vi "U3 Create Frequency Output Lists.vi"() -> (1 "Period List":dbl[][](array[numeric]) format="%.6f", 2 "Frequency List":dbl[][](array[numeric]) format="%.6f")   [LabVIEW 2021]
panel:
  # "Creates 2D arrays which are lists of all the frequency/period\noptions for the Frequency Output timer mode 7.  Takes 10-15\nseconds to run on a typical PC.\n\nFrequency/Period, Base Clock, Divisor, Timer Value"
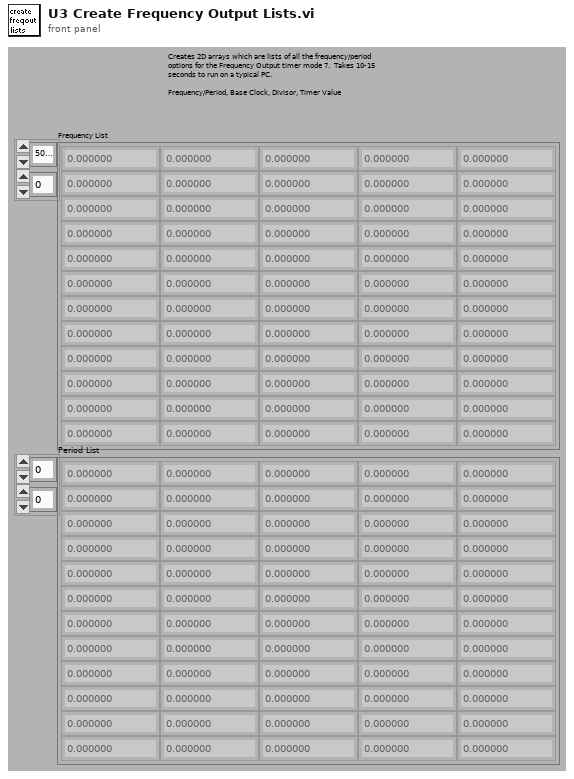
[diagram p1: front panel]
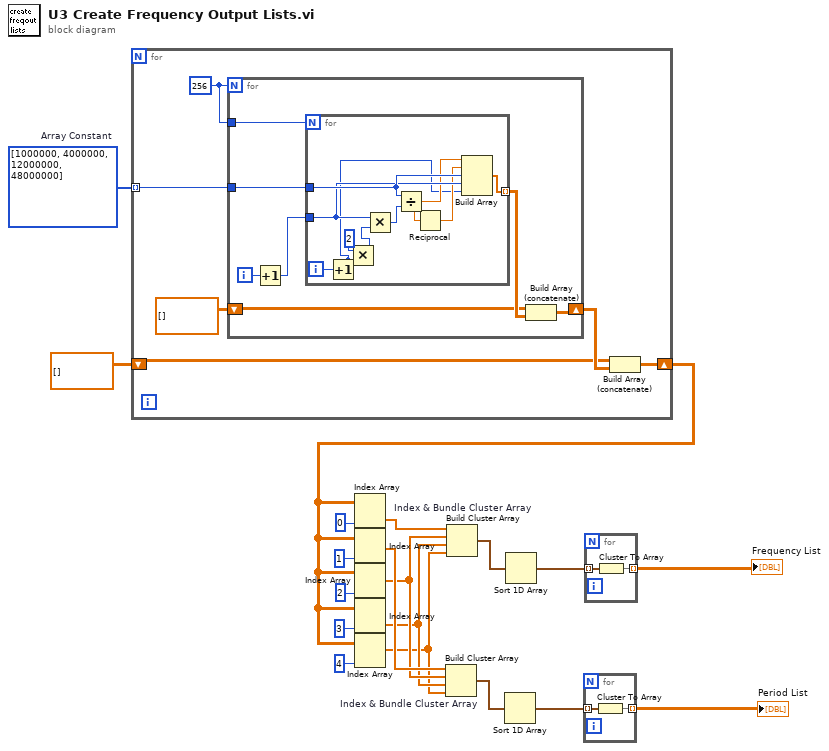
[diagram p0: block diagram]
diagram:
  w17 = i32[] [1000000, 4000000, 12000000, 48000000]  # Array Constant
  n1 = for {
    tunnel: w17 -> [w25] mode=indexing
    shift-right: [w21] -> w8
    shift-left: dbl[][] [] -> [w22]
    w24 = 256
    n2 = for {
      N: w24 -> [_]
      tunnel: w25 -> [w32]
      tunnel: w24 -> [w31]
      shift-right: [w26] -> w23
      shift-left: dbl[][] [] -> [w27]
      i -> [w30]
      n3 = Increment(x=w30) -> (x+1=w29:i32)
      n4 = for {
        N: w31 -> [_]
        tunnel: w32 -> [w40]
        tunnel: w29 -> [w39]
        tunnel: [w38] -> w28 mode=indexing
        i -> [w42]
        n5 = Increment(x=w42) -> (x+1=w33:i32)
        n6 = Multiply(x=2, y=w33) -> (x*y=w34:i32)
        n7 = Multiply(x=w39, y=w34) -> (x*y=w41:i32)
        n8 = Divide(x=w40, y=w41) -> (x/y=w36:dbl)
        n9 = Reciprocal(x=w36) -> (1/x=w35:dbl)
        n10 = Build Array(w36, w35, w40, w39, w33) -> (w38:dbl[])
      }
      n11 = Build Array (concatenate)(w27, w28) -> (w26:dbl[][])
    }
    n12 = Build Array (concatenate)(w22, w23) -> (w21:dbl[][])
  }
  n13 = Index Array(array=w8, index (col)=0) -> (element=w15:dbl[])  [unwired: 1 in]
  n14 = Index Array(array=w8, index (col)=1) -> (element=w4:dbl[])  [unwired: 1 in]
  n15 = Index Array(array=w8, index (col)=2) -> (element=w3:dbl[])  [unwired: 1 in]
  n16 = Index Array(array=w8, index (col)=3) -> (element=w2:dbl[])  [unwired: 1 in]
  n17 = Index Array(array=w8, index (col)=4) -> (element=w1:dbl[])  [unwired: 1 in]
  n18 = Build Cluster Array "Index & Bundle Cluster Array"(w4, w3, w2, w1) -> (w5:cluster{dbl, dbl, dbl, dbl}[])
  n19 = Build Cluster Array "Index & Bundle Cluster Array"(w15, w3, w2, w1) -> (w14:cluster{dbl, dbl, dbl, dbl}[])
  n20 = Sort 1D Array(array=w5) -> (sorted array=w6:cluster{dbl, dbl, dbl, dbl}[])
  n21 = Sort 1D Array(array=w14) -> (sorted array=w13:cluster{dbl, dbl, dbl, dbl}[])
  n22 = for {
    tunnel: w6 -> [w44] mode=indexing
    tunnel: [w43] -> w18 mode=indexing
    n23 = Cluster To Array(cluster=w44) -> (array=w43:dbl[])
  }
  "Period List" <- w18
  n24 = for {
    tunnel: w13 -> [w46] mode=indexing
    tunnel: [w45] -> w19 mode=indexing
    n25 = Cluster To Array(cluster=w46) -> (array=w45:dbl[])
  }
  "Frequency List" <- w19
